vi "Documentation.vi"   [LabVIEW 2019, in "Inst.Framework-Template.lvclass"]
uses:
  Inst.Framework-Template.lvclass
  9169cc93-ed84-4232-9f90-6ee16c7bb454.vi
  de41cf0e-ff2b-4a51-852c-55dbec0e345b.vi
  9169cc93-ed84-4232-9f90-6ee16c7bb454.vi/3bc1a7ce-2052-4bb6-955b-7b4bb15f1b3f.vi
  de41cf0e-ff2b-4a51-852c-55dbec0e345b.vi/21da6090-1418-40bf-b1d0-aaaa039838a5.vi
  9169cc93-ed84-4232-9f90-6ee16c7bb454.vi/3bc1a7ce-2052-4bb6-955b-7b4bb15f1b3f.vi/186c7484-df9a-4054-807c-655d760e15c8.vi
  <userlib>/LevyLab/Instrument Framework/SMOs/Instrument/API/Send and Receive.vi
  9169cc93-ed84-4232-9f90-6ee16c7bb454.vi/3bc1a7ce-2052-4bb6-955b-7b4bb15f1b3f.vi/d68663b6-9a59-49ac-8a3e-6c41418329a1.vi
  <userlib>/LevyLab/Instrument Framework/SMOs/Instrument/Private/Get Client Type.vi
  de41cf0e-ff2b-4a51-852c-55dbec0e345b.vi/21da6090-1418-40bf-b1d0-aaaa039838a5.vi/9c6ae891-6b7b-494d-b8a3-540145664cba.vi
  de41cf0e-ff2b-4a51-852c-55dbec0e345b.vi/21da6090-1418-40bf-b1d0-aaaa039838a5.vi/557a546d-74cb-4577-b055-fbd1aae73a04.vi
  9169cc93-ed84-4232-9f90-6ee16c7bb454.vi/3bc1a7ce-2052-4bb6-955b-7b4bb15f1b3f.vi/186c7484-df9a-4054-807c-655d760e15c8.vi/d1b53759-cdad-4b30-913c-d0af3a047282.vi
  9169cc93-ed84-4232-9f90-6ee16c7bb454.vi/3bc1a7ce-2052-4bb6-955b-7b4bb15f1b3f.vi/186c7484-df9a-4054-807c-655d760e15c8.vi/7fe9f392-2cd1-45ec-9a03-6ef05e8253b6.vi
  9169cc93-ed84-4232-9f90-6ee16c7bb454.vi/3bc1a7ce-2052-4bb6-955b-7b4bb15f1b3f.vi/d68663b6-9a59-49ac-8a3e-6c41418329a1.vi/8fac68c8-b375-4435-9af1-ae7d05afa959.vi
  9169cc93-ed84-4232-9f90-6ee16c7bb454.vi/3bc1a7ce-2052-4bb6-955b-7b4bb15f1b3f.vi/d68663b6-9a59-49ac-8a3e-6c41418329a1.vi/1362d31b-bfc4-4d78-893d-5589c90f5b2b.vi
  de41cf0e-ff2b-4a51-852c-55dbec0e345b.vi/21da6090-1418-40bf-b1d0-aaaa039838a5.vi/9c6ae891-6b7b-494d-b8a3-540145664cba.vi/19fa3c45-0d16-4bb0-b2ad-138c00be1b64.vi
  de41cf0e-ff2b-4a51-852c-55dbec0e345b.vi/21da6090-1418-40bf-b1d0-aaaa039838a5.vi/9c6ae891-6b7b-494d-b8a3-540145664cba.vi/55c769c2-5611-4ccb-aecc-8b538907d375.vi
  de41cf0e-ff2b-4a51-852c-55dbec0e345b.vi/21da6090-1418-40bf-b1d0-aaaa039838a5.vi/557a546d-74cb-4577-b055-fbd1aae73a04.vi/b0531fe4-9e29-4687-baa2-aadea3dcdf03.vi
  de41cf0e-ff2b-4a51-852c-55dbec0e345b.vi/21da6090-1418-40bf-b1d0-aaaa039838a5.vi/557a546d-74cb-4577-b055-fbd1aae73a04.vi/d5c1aeff-1834-4139-868c-d1c2b7ad11df.vi
  9169cc93-ed84-4232-9f90-6ee16c7bb454.vi/3bc1a7ce-2052-4bb6-955b-7b4bb15f1b3f.vi/d68663b6-9a59-49ac-8a3e-6c41418329a1.vi/8fac68c8-b375-4435-9af1-ae7d05afa959.vi/29d737dc-f0a6-4278-8ea1-10f2043af5e9.vi
  9169cc93-ed84-4232-9f90-6ee16c7bb454.vi/3bc1a7ce-2052-4bb6-955b-7b4bb15f1b3f.vi/d68663b6-9a59-49ac-8a3e-6c41418329a1.vi/8fac68c8-b375-4435-9af1-ae7d05afa959.vi/10a74567-eb18-4897-8559-1a35f16d5028.vi
  de41cf0e-ff2b-4a51-852c-55dbec0e345b.vi/21da6090-1418-40bf-b1d0-aaaa039838a5.vi/557a546d-74cb-4577-b055-fbd1aae73a04.vi/b0531fe4-9e29-4687-baa2-aadea3dcdf03.vi/aeda4fc1-3546-460b-8fa5-afdc0bea1e87.vi
  de41cf0e-ff2b-4a51-852c-55dbec0e345b.vi/21da6090-1418-40bf-b1d0-aaaa039838a5.vi/557a546d-74cb-4577-b055-fbd1aae73a04.vi/b0531fe4-9e29-4687-baa2-aadea3dcdf03.vi/ed5f9993-61e6-48eb-895f-b725d41d8077.vi
  <userlib>/LevyLab/Instrument Framework/SMOs/Instrument/Private/Get RC Connection Status.vi
  <userlib>/LevyLab/Instrument Framework/SMOs/Instrument/API/Enum to String.vi
  <userlib>/LevyLab/Instrument Framework/SMOs/RemoteControl/API/Send and Receive.vi
  <vilib>/Utility/Data Type/Get Type Information.vi
  <vilib>/JDP Science/JSONtext/JSON text to Variant.vi
  <userlib>/LevyLab/Instrument Framework/SMOs/Instrument/API/Instrument.GetPublicEvents.vi
  <vilib>/JDP Science/JSONtext/Variant to JSON Text.vi
  <vilib>/National Instruments/GUID Generator/Guid Generator.vi
  <userlib>/LevyLab/Instrument Framework/SMOs/Instrument/Private/Instrument.MessageFromProcess.EventStructure.vi
  <userlib>/LevyLab/Instrument Framework/SMOs/Instrument/Instrument.lvclass
  <vilib>/JKI/JKI SMO/SMO/SMO.lvclass
  Typedefs/Inst.Framework-Template.Commands--Enum.ctl
  Typedefs/Inst.Framework-Template.getAll--Cluster.ctl
  Typedefs/Inst.Framework-Template.Configuration--Cluster.ctl
  Inst UI.Framework-Template/Inst UI.Framework-Template.lvclass
  <vilib>/JDP Science/JSONtext/LVClass Serializer/JSONtext LVClass Serializer.lvclass
  Inst UI.Framework-Template/Inst UI.Framework-Template.UI--Cluster.ctl
  <userlib>/LevyLab/Instrument Framework/SMOs/Instrument UI/Instrument UI.lvclass
  <vilib>/JKI/JKI SMO/SMO.UI/SMO.UI.lvclass
  C:/Program Files (x86)/National Instruments/LabVIEW 2019/vi.lib/JKI/JKI SMO/SMO/SMO.lvclass
  C:/Program Files (x86)/National Instruments/LabVIEW 2019/user.lib/LevyLab/Instrument Framework/SMOs/Instrument/Instrument.lvclass
  C:/Program Files (x86)/National Instruments/LabVIEW 2019/user.lib/LevyLab/Instrument Framework/SMOs/Instrument UI/Instrument UI.lvclass
  C:/Program Files (x86)/National Instruments/LabVIEW 2019/vi.lib/JKI/JKI SMO/SMO.UI/SMO.UI.lvclass
types:
  T1 = typedef "Inst.Framework-Template.lvclass/Inst.Framework-Template.Configuration--Cluster.ctl" = cluster{"Example Setting 1":dbl, "Example Setting 2":dbl, "Example Setting 3":string}
  T2 = typedef "Inst.Framework-Template.lvclass/Inst.Framework-Template.getAll--Cluster.ctl" = cluster{"Levy 1":dbl, "Logger SMO":dbl, "SMO Boolean":bool, "SMO String":string}
  T3 = typedef "Inst.Framework-Template.lvclass/Inst.Framework-Template.Commands--Enum.ctl" = enum16{"Do Something"}
  T4 = typedef "Inst UI.Framework-Template.lvclass/Inst UI.Framework-Template.UI--Cluster.ctl" = cluster{"Parameter":dbl, "Parameter 2":string}
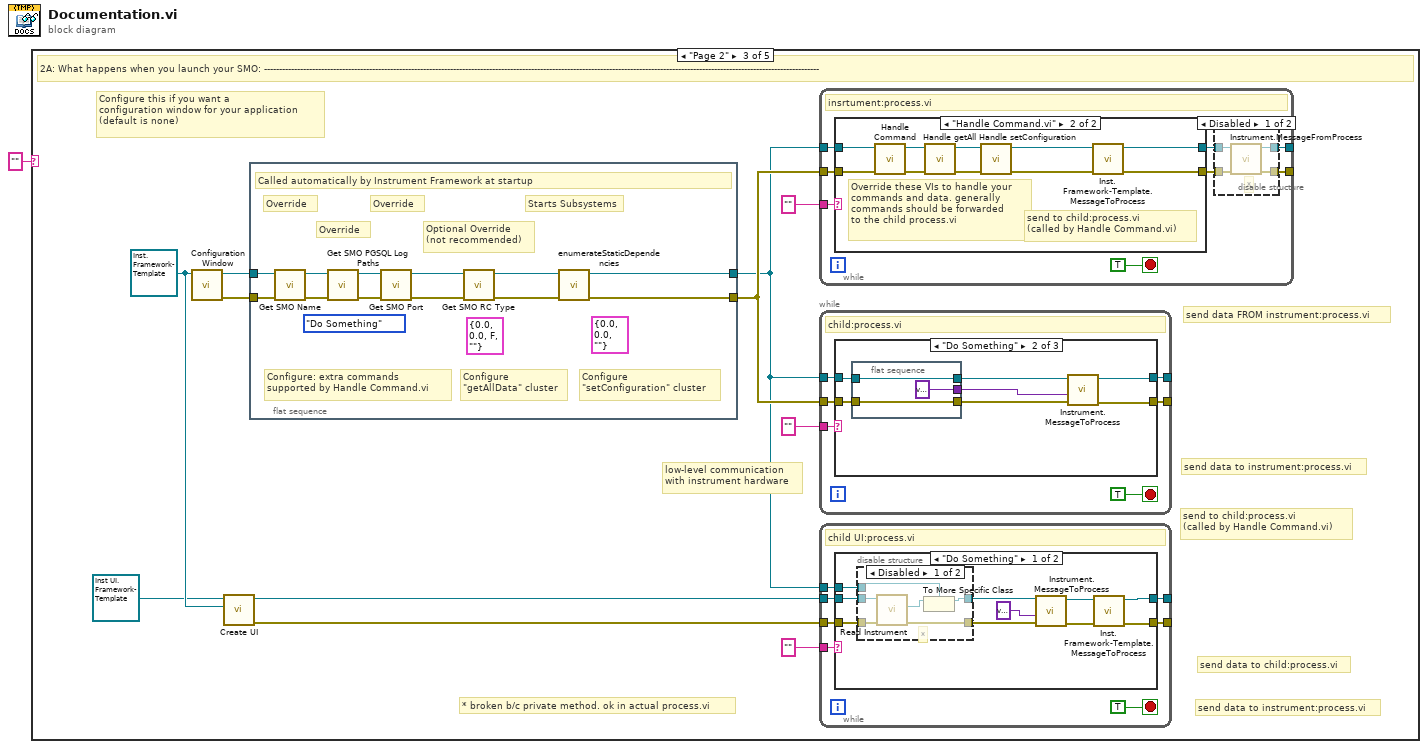
[diagram p0: block diagram]
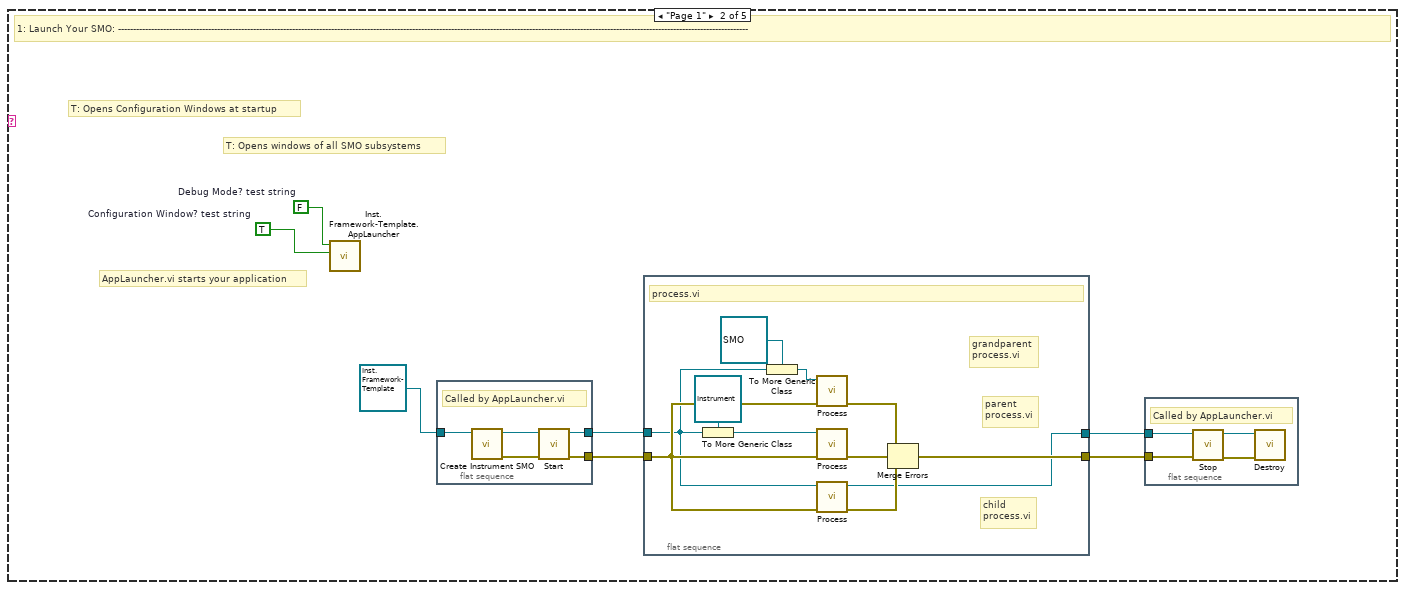
[diagram p3: hidden frame]
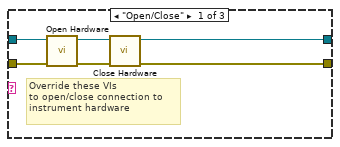
[diagram p6: hidden frame]
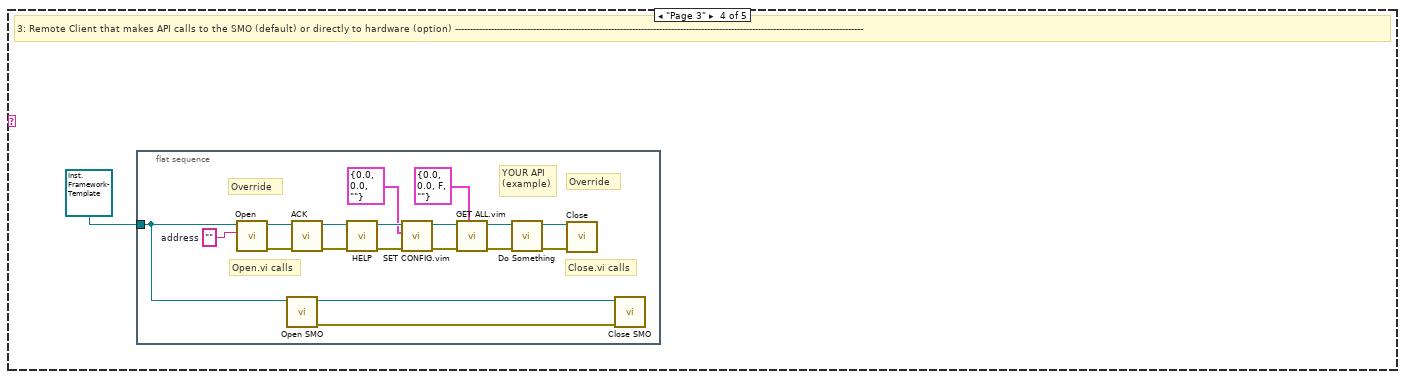
[diagram p10: hidden frame]
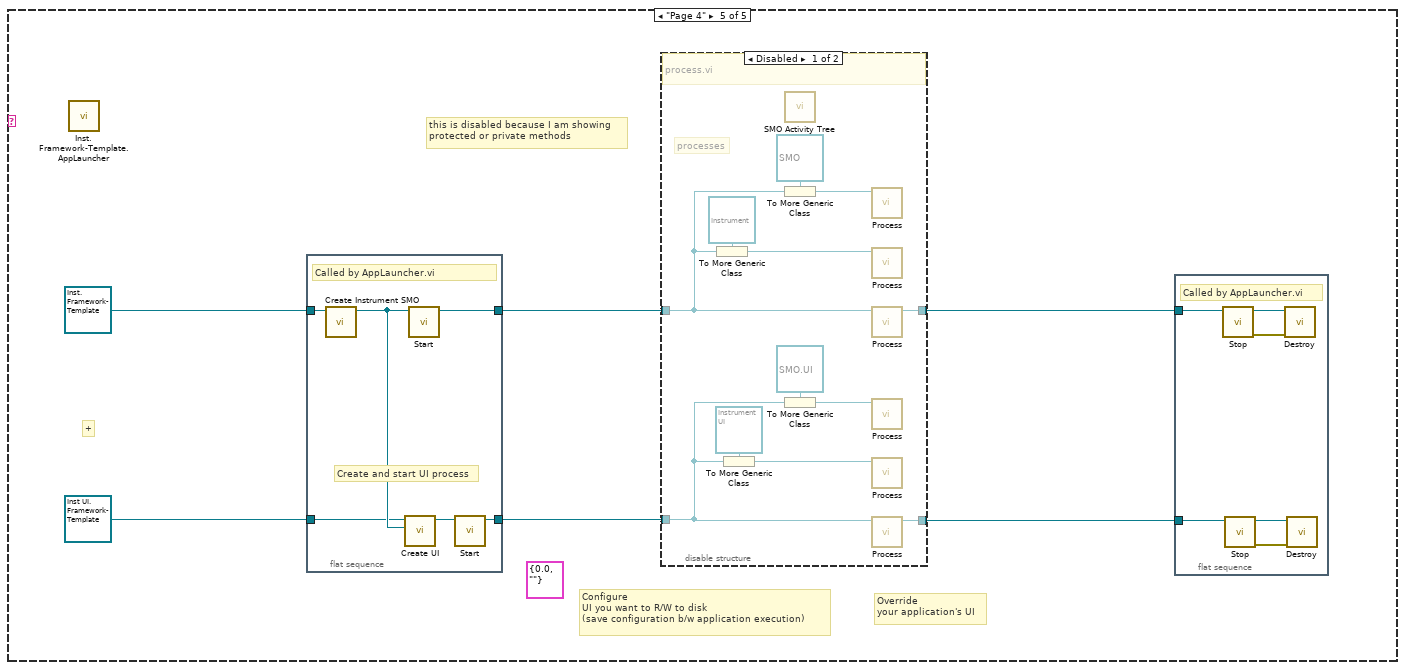
[diagram p11: hidden frame]
diagram:
  n1 = case shown="\"Page 2\"" "" {
    frame Default {
    }
    frame "Page 1" {
      w7 = TRUE  # Configuration Window? test string
      w8 = FALSE  # Debug Mode? test string
      # "AppLauncher.vi starts your application"
      # "T: Opens windows of all SMO subsystems"
      # "T: Opens Configuration Windows at startup"
      # "1: Launch Your SMO: ------------------------------------------------------------------------------------------------------------------------------------------------------------------------------------------------------------------"
      n2 = call "Inst.Framework-Template.AppLauncher.vi"("Config Window"=w7, "Debug Mode"=w8) -> ()  [unwired: 9 in, 1 out]
      n3 = flat-sequence {
        tunnel: [w26] -> w3
        tunnel: [w25] -> w5
        tunnel: refnum<class "Inst.Framework-Template.lvclass"> refnum ("Instrument.Template.lvclass") -> [w24]
        frame #0 {
          # "Called by AppLauncher.vi"
          n4 = call-dynamic "Create Instrument SMO.vi"("Instrument in"=w24) -> ("error out"=w27:errorcluster, "Instrument out"=w28:refnum<class "Inst.Framework-Template.lvclass">)  [unwired: 9 in]
          n5 = call <vilib>:"Start.vi"("error in (no error)"=w27, "SMO"=w28) -> ("error out"=w25:errorcluster, "SMO out"=w26:refnum<class "Inst.Framework-Template.lvclass">)  [unwired: 8 in]
        }
      }
      n6 = flat-sequence {
        tunnel: [w19] -> w6
        tunnel: w5 -> [w17]
        tunnel: [w11] -> w4
        tunnel: w3 -> [w10]
        frame #0 {
          # "child\nprocess.vi"
          # "grandparent\nprocess.vi"
          # "parent\nprocess.vi"
          # "process.vi"
          n7 = To More Generic Class(target class=refnum<class "Instrument.lvclass"> refnum ("Instrument"), reference=w10) -> (generic class reference=w16:refnum<class "Instrument.lvclass">)
          n8 = To More Generic Class(target class=refnum<class "SMO.lvclass"> refnum ("SMO"), reference=w10) -> (generic class reference=w18:refnum<class "SMO.lvclass">)
          n9 = call-dynamic "Process.vi"("error in"=w17, "SMO"=w18) -> ("error out"=w12:errorcluster)  [unwired: 8 in, 1 out]
          n10 = call-dynamic "Process.vi"("error in"=w17, "Instrument"=w16) -> ("error out"=w14:errorcluster)  [unwired: 8 in, 1 out]
          n11 = call-dynamic "Process.vi"("error in"=w17, "Framework-Template"=w10) -> ("error out"=w13:errorcluster, "Framework-Template out"=w11:refnum<class "Inst.Framework-Template.lvclass">)  [unwired: 8 in]
          n12 = Merge Errors(w12, w14, w13) -> (w19:errorcluster)
        }
      }
      n13 = flat-sequence {
        tunnel: w4 -> [w21]
        tunnel: w6 -> [w20]
        frame #0 {
          # "Called by AppLauncher.vi"
          n14 = call <vilib>:"Stop.vi"("error in (no error)"=w20, "SMO"=w21) -> ("error out"=w23:errorcluster, "SMO out"=w22:refnum<class "Inst.Framework-Template.lvclass">)  [unwired: 8 in]
          n15 = call <vilib>:"Destroy.vi"("error in (no error)"=w23, "SMO"=w22) -> ()  [unwired: 9 in, 1 out]
        }
      }
    }
    frame "Page 2" {
      w34 = refnum<class "Inst.Framework-Template.lvclass"> refnum ("Instrument.Template.lvclass")
      # "send data FROM instrument:process.vi"
      # "send data to child:process.vi"
      # "send to child:process.vi\n(called by Handle Command.vi)"
      # "* broken b/c private method. ok in actual process.vi"
      # "send data to instrument:process.vi"
      # "low-level communication\nwith instrument hardware"
      # "send data to instrument:process.vi"
      # "Configure this if you want a\nconfiguration window for your application\n(default is none)"
      # "2A: What happens when you launch your SMO: -----------------------------------------------------------------------------------------------------------------------------------------------------------------------------------------"
      n16 = call-dynamic "Configuration Window.vi"("Inst.Framework-Template in"=w34) -> ("error out"=w38:errorcluster, "Inst.Framework-Template out"=w39:refnum<class "Inst.Framework-Template.lvclass">)  [unwired: 9 in]
      n17 = call <userlib>:"Create UI.vi"("Instrument in"=w34, "Instrument UI"=refnum<class "Inst UI.Framework-Template.lvclass"> refnum ("Instrument UI.Template.lvclass")) -> ("error out"=w31:errorcluster, "Instrument UI out"=w32:refnum<class "Inst UI.Framework-Template.lvclass">)  [unwired: 8 in]
      n18 = flat-sequence {
        tunnel: w39 -> [w121]
        tunnel: w38 -> [w116]
        tunnel: [w115] -> w35
        tunnel: [w114] -> w29
        frame #0 {
          (unwired) T1 {"Example Setting 1"=0.0, "Example Setting 2"=0.0, "Example Setting 3"=""} ("Configuration")
          (unwired) T2 {"Levy 1"=0.0, "Logger SMO"=0.0, "SMO Boolean"=FALSE, "SMO String"=""} ("getAll")
          (unwired) Inst.Framework-Template.Commands--Enum."Do Something" ("Commands")
          # "Configure\n\"setConfiguration\" cluster"
          # "Configure\n\"getAllData\" cluster"
          # "Configure: extra commands\nsupported by Handle Command.vi"
          # "Starts Subsystems"
          # "Override"
          # "Override"
          # "Override"
          # "Optional Override\n(not recommended)"
          # "Called automatically by Instrument Framework at startup"
          n19 = call-dynamic "Get SMO Name.vi"("error in (no error)"=w116, "Inst.Framework-Template in"=w121) -> ("error out"=w119:errorcluster, "Inst.Framework-Template out"=w120:refnum<class "Inst.Framework-Template.lvclass">)  [unwired: 7 in, 1 out]
          n20 = call-dynamic "Get SMO PGSQL Log Paths.vi"("error in (no error)"=w119, "Inst.Framework-Template in"=w120) -> ("error out"=w117:errorcluster, "Inst.Framework-Template out"=w118:refnum<class "Inst.Framework-Template.lvclass">)  [unwired: 7 in, 1 out]
          n21 = call-dynamic "Get SMO Port.vi"("error in (no error)"=w117, "Inst.Framework-TemplateInstrument in"=w118) -> ("error out"=w122:errorcluster, "Inst.Framework-TemplateInstrument out"=w123:refnum<class "Inst.Framework-Template.lvclass">)  [unwired: 7 in, 1 out]
          n22 = call-dynamic "Get SMO RC Type.vi"("error in (no error)"=w122, "Inst.Framework-TemplateInstrument in"=w123) -> ("error out"=w124:errorcluster, "Inst.Framework-TemplateInstrument out"=w125:refnum<class "Inst.Framework-Template.lvclass">)  [unwired: 7 in, 1 out]
          n23 = call-dynamic "enumerateStaticDependencies.vi"("error in (no error)"=w124, "Instrument"=w125) -> ("error out"=w115:errorcluster, "Instrument out"=w114:refnum<class "Inst.Framework-Template.lvclass">)  [unwired: 7 in, 1 out]
        }
      }
      n24 = while {
        tunnel: "" -> [w97]
        tunnel: w29 -> [w95]
        tunnel: [w90] -> _
        tunnel: w35 -> [w94]
        tunnel: [w91] -> _
        stop <- TRUE stop-if-true
        # "insrtument:process.vi"
        n25 = case shown="\"Handle Command.vi\"" w97 {
          tunnel: w95 -> [w103 w113]
          tunnel: [w103 w106] -> w93
          tunnel: w94 -> [w102 w112]
          tunnel: [w102 w105] -> w92
          frame Default {
          }
          frame "Handle Command.vi" {
            # "send to child:process.vi\n(called by Handle Command.vi)"
            # "Override these VIs to handle your\ncommands and data. generally \ncommands should be forwarded\nto the child process.vi"
            n26 = call-dynamic "Handle Command.vi"("error in (no error)"=w112, "Inst.Framework-Template in"=w113) -> ("error out"=w108:errorcluster, "Inst.Framework-Template out"=w111:refnum<class "Inst.Framework-Template.lvclass">)  [unwired: 6 in, 2 out]
            n27 = call-dynamic "Handle getAll.vi"("error in (no error)"=w108, "Inst.Framework-Template in"=w111) -> ("error out"=w109:errorcluster, "Inst.Framework-Template out"=w110:refnum<class "Inst.Framework-Template.lvclass">)  [unwired: 7 in, 1 out]
            n28 = call-dynamic "Handle setConfiguration.vi"("error in (no error)"=w109, "Inst.Framework-Template in"=w110) -> ("error out"=w104:errorcluster, "Inst.Framework-Template out"=w107:refnum<class "Inst.Framework-Template.lvclass">)  [unwired: 8 in]
            n29 = call "Inst.Framework-Template.MessageToProcess.vi"("error in (no error)"=w104, "Framework-Template in"=w107) -> ("error out"=w105:errorcluster, "Framework-Template out"=w106:refnum<class "Inst.Framework-Template.lvclass">)  [unwired: 8 in]
          }
        }
        n30 = disable-structure shown="Disabled" {
          disable-tunnel: w93 -> [w101 _]
          disable-tunnel: w92 -> [w100 _]
          disable-tunnel: [w99 _] -> w91
          disable-tunnel: [w98 _] -> w90
          frame Disabled {
            # "*"
            n31 = call <userlib>:"Instrument.MessageFromProcess.vi"("error in (no error)"=w100, "Instrument"=w101) -> ("error out"=w99:errorcluster, "Instrument out"=w98:refnum<class "Inst.Framework-Template.lvclass">)  [unwired: 8 in]
          }
          frame Enabled {
          }
        }
      }
      n32 = while {
        tunnel: "" -> [w71]
        tunnel: w29 -> [w69]
        tunnel: [w68] -> _
        tunnel: w35 -> [w67]
        tunnel: [w66] -> _
        stop <- TRUE stop-if-true
        # "child:process.vi"
        n33 = case shown="\"Do Something\"" w71 {
          tunnel: w69 -> [w74 w80 w89]
          tunnel: [w73 w84 w89] -> w68
          tunnel: w67 -> [w77 w82 w88]
          tunnel: [w72 w83 w88] -> w66
          frame "Open/Close" {
            # "Override these VIs\nto open/close connection to\ninstrument hardware"
            n34 = call-dynamic "Open Hardware.vi"("error in (no error)"=w77, "Inst.Framework-Template in"=w74) -> ("error out"=w76:errorcluster, "Inst.Framework-Template out"=w75:refnum<class "Inst.Framework-Template.lvclass">)  [unwired: 8 in]
            n35 = call-dynamic "Close Hardware.vi"("error in (no error)"=w76, "Inst.Framework-Template in"=w75) -> ("error out"=w72:errorcluster, "Inst.Framework-Template out"=w73:refnum<class "Inst.Framework-Template.lvclass">)  [unwired: 8 in]
          }
          frame "Do Something" {
            n36 = flat-sequence {
              tunnel: w82 -> [w87]
              tunnel: [w87] -> w81
              tunnel: w80 -> [w86]
              tunnel: [w86] -> w79
              tunnel: [variant ("Data")] -> w78
              frame #0 {
              }
            }
            n37 = call <userlib>:"Instrument.MessageToProcess.vi"("error in (no error)"=w81, "Data"=w78, "Instrument"=w79) -> ("error out"=w83:errorcluster, "Instrument out"=w84:refnum<class "Inst.Framework-Template.lvclass">)  [unwired: 7 in]
          }
          frame Default {
          }
        }
      }
      n38 = while {
        tunnel: "" -> [w46]
        tunnel: w32 -> [w44]
        tunnel: [w43] -> _
        tunnel: w31 -> [w42]
        tunnel: [w41] -> _
        tunnel: w29 -> [w40]
        stop <- TRUE stop-if-true
        # "child UI:process.vi"
        n39 = case shown="\"Do Something\"" w46 {
          tunnel: w44 -> [w55 _]
          tunnel: [w49 w64] -> w43
          tunnel: w42 -> [w56 w65]
          tunnel: [w48 w65] -> w41
          tunnel: w40 -> [w51 w64]
          frame "Do Something" {
            # "*"
            n40 = disable-structure shown="Disabled" {
              disable-tunnel: w56 -> [w62 _]
              disable-tunnel: w55 -> [w61 _]
              disable-tunnel: [w60 _] -> w54
              disable-tunnel: w51 -> [w58 w63]
              disable-tunnel: [w57 w63] -> w50
              frame Disabled {
                n41 = call <userlib>:"Read Instrument.vi"("error in (no error)"=w62, "Instrument UI in"=w61) -> ("error out"=w60:errorcluster, "Instrument"=w59:refnum<class "Instrument.lvclass">)  [unwired: 7 in, 1 out]
                n42 = To More Specific Class(target class=w58, reference=w59) -> (specific class reference=w57:refnum<class "Inst.Framework-Template.lvclass">)  [unwired: 1 in, 1 out]
              }
              frame Enabled {
              }
            }
            n43 = call <userlib>:"Instrument.MessageToProcess.vi"("error in (no error)"=w54, "Data"=variant, "Instrument"=w50) -> ("error out"=w47:errorcluster, "Instrument out"=w52:refnum<class "Inst.Framework-Template.lvclass">)  [unwired: 7 in]
            n44 = call "Inst.Framework-Template.MessageToProcess.vi"("error in (no error)"=w47, "Framework-Template in"=w52) -> ("error out"=w48:errorcluster, "Framework-Template out"=w49:refnum<class "Inst.Framework-Template.lvclass">)  [unwired: 8 in]
          }
          frame Default {
          }
        }
      }
    }
    frame "Page 3" {
      # "3: Remote Client that makes API calls to the SMO (default) or directly to hardware (option) ----------------------------------------------------------------------------------------------------------------------------------------"
      n45 = flat-sequence {
        tunnel: refnum<class "Inst.Framework-Template.lvclass"> refnum ("Instrument.Template.lvclass") -> [w127]
        frame #0 {
          w130 = ""  # address
          # "Close.vi calls"
          # "Open.vi calls"
          # "YOUR API\n(example)"
          # "Override"
          # "Override"
          n46 = call-dynamic "Open.vi"("address"=w130, "Inst.Framework-Template in"=w127) -> ("error out"=w144:errorcluster, "Inst.Framework-Template out"=w143:refnum<class "Inst.Framework-Template.lvclass">)  [unwired: 8 in]
          n47 = call <userlib>:"Open SMO.vi"("Instrument in"=w127) -> ("error out"=w128:errorcluster, "Instrument out"=w129:refnum<class "Inst.Framework-Template.lvclass">)  [unwired: 9 in]
          n48 = call <userlib>:"ACK.vi"("error in (no error)"=w144, "Instrument in"=w143) -> ("error out"=w142:errorcluster, "Instrument out"=w141:refnum<class "Inst.Framework-Template.lvclass">)  [unwired: 7 in, 1 out]
          n49 = call <userlib>:"HELP.vi"("error in (no error)"=w142, "Instrument in"=w141) -> ("error out"=w136:errorcluster, "Instrument in"=w137:refnum<class "Inst.Framework-Template.lvclass">)  [unwired: 7 in, 1 out]
          n50 = call "SET CONFIG.vim"("error in (no error)"=w136, "Configuration"=T1 {"Example Setting 1"=0.0, "Example Setting 2"=0.0, "Example Setting 3"=""}, "Instrument in"=w137) -> ("error out"=w131:errorcluster, "Instrument out"=w134:refnum<class "Inst.Framework-Template.lvclass">)  [unwired: 7 in]
          n51 = call "GET ALL.vim"("type"=T2 {"Levy 1"=0.0, "Logger SMO"=0.0, "SMO Boolean"=FALSE, "SMO String"=""} ("getAll"), "error in (no error)"=w131, "Instrument in"=w134) -> ("error out"=w132:errorcluster, "Instrument out"=w133:refnum<class "Inst.Framework-Template.lvclass">)  [unwired: 6 in, 1 out]
          n52 = call-dynamic "Do Something.vi"("error in (no error)"=w132, "Inst.Framework-Template in"=w133) -> ("error out"=w139:errorcluster, "Inst.Framework-Template out"=w140:refnum<class "Inst.Framework-Template.lvclass">)  [unwired: 8 in]
          n53 = call-dynamic "Close.vi"("error in (no error)"=w139, "Inst.Framework-Template in"=w140) -> ()  [unwired: 8 in, 2 out]
          n54 = call <userlib>:"Close SMO.vi"("error in (no error)"=w128, "Instrument in"=w129) -> ()  [unwired: 8 in, 2 out]
        }
      }
    }
    frame "Page 4" {
      (unwired) T4 {"Parameter"=0.0, "Parameter 2"=""} ("UI")
      # "this is disabled because I am showing\nprotected or private methods"
      # "Configure\nUI you want to R/W to disk\n(save configuration b/w application execution)"
      # "Override\nyour application's UI"
      # "+"
      n55 = call "Inst.Framework-Template.AppLauncher.vi"() -> ()  [unwired: 11 in, 1 out]
      n56 = flat-sequence {
        tunnel: [w162] -> w148
        tunnel: refnum<class "Inst.Framework-Template.lvclass"> refnum ("Instrument.Template.lvclass") -> [w161]
        tunnel: refnum<class "Inst UI.Framework-Template.lvclass"> refnum ("Instrument UI.Template.lvclass") -> [w159]
        tunnel: [w157] -> w146
        frame #0 {
          # "Create and start UI process"
          # "Called by AppLauncher.vi"
          n57 = call-dynamic "Create Instrument SMO.vi"("Instrument in"=w161) -> ("Instrument out"=w160:refnum<class "Inst.Framework-Template.lvclass">)  [unwired: 9 in, 1 out]
          n58 = call <userlib>:"Create UI.vi"("Instrument in"=w160, "Instrument UI"=w159) -> ("Instrument UI out"=w158:refnum<class "Inst UI.Framework-Template.lvclass">)  [unwired: 8 in, 1 out]
          n59 = call <vilib>:"Start.vi"("SMO"=w160) -> ("SMO out"=w162:refnum<class "Inst.Framework-Template.lvclass">)  [unwired: 9 in, 1 out]
          n60 = call <vilib>:"Start.vi"("SMO"=w158) -> ("SMO out"=w157:refnum<class "Inst UI.Framework-Template.lvclass">)  [unwired: 9 in, 1 out]
        }
      }
      n61 = disable-structure shown="Disabled" {
        disable-tunnel: [w174 w176] -> w149
        disable-tunnel: w148 -> [w173 w176]
        disable-tunnel: w146 -> [w172 w175]
        disable-tunnel: [w171 w175] -> w145
        frame Disabled {
          # "processes"
          # "process.vi"
          n62 = To More Generic Class(target class=refnum<class "Instrument.lvclass"> refnum ("Instrument"), reference=w173) -> (generic class reference=w169:refnum<class "Instrument.lvclass">)
          n63 = To More Generic Class(target class=refnum<class "Instrument UI.lvclass"> refnum ("Instrument UI"), reference=w172) -> (generic class reference=w165:refnum<class "Instrument UI.lvclass">)
          n64 = call <vilib>:"SMO Activity Tree.vi"() -> ()  [unwired: 12 in]
          n65 = To More Generic Class(target class=refnum<class "SMO.lvclass"> refnum ("SMO"), reference=w173) -> (generic class reference=w170:refnum<class "SMO.lvclass">)
          n66 = To More Generic Class(target class=refnum<class "SMO.UI.lvclass"> refnum ("SMO.UI"), reference=w172) -> (generic class reference=w163:refnum<class "SMO.UI.lvclass">)
          n67 = call-dynamic "Process.vi"("SMO"=w170) -> ()  [unwired: 9 in, 2 out]
          n68 = call-dynamic "Process.vi"("Instrument"=w169) -> ()  [unwired: 9 in, 2 out]
          n69 = call-dynamic "Process.vi"("Framework-Template"=w173) -> ("Framework-Template out"=w174:refnum<class "Inst.Framework-Template.lvclass">)  [unwired: 9 in, 1 out]
          n70 = call-dynamic "Process.vi"("SMO.UI"=w163) -> ()  [unwired: 9 in, 2 out]
          n71 = call-dynamic "Process.vi"("Instrument UI in"=w165) -> ()  [unwired: 9 in, 2 out]
          n72 = call-dynamic "Process.vi"("Inst UI.Framework-Template"=w172) -> ("Inst UI.Framework-Template out"=w171:refnum<class "Inst UI.Framework-Template.lvclass">)  [unwired: 9 in, 1 out]
        }
        frame Enabled {
        }
      }
      n73 = flat-sequence {
        tunnel: w149 -> [w154]
        tunnel: w145 -> [w152]
        frame #0 {
          # "Called by AppLauncher.vi"
          n74 = call <vilib>:"Stop.vi"("SMO"=w154) -> ("error out"=w156:errorcluster, "SMO out"=w155:refnum<class "Inst.Framework-Template.lvclass">)  [unwired: 9 in]
          n75 = call <vilib>:"Stop.vi"("SMO"=w152) -> ("error out"=w153:errorcluster, "SMO out"=w151:refnum<class "Inst UI.Framework-Template.lvclass">)  [unwired: 9 in]
          n76 = call <vilib>:"Destroy.vi"("error in (no error)"=w156, "SMO"=w155) -> ()  [unwired: 9 in, 1 out]
          n77 = call <vilib>:"Destroy.vi"("error in (no error)"=w153, "SMO"=w151) -> ()  [unwired: 9 in, 1 out]
        }
      }
    }
  }
